vi "Set Auxiliary Amplifier Mode.vi"(8 "error in (no error)":errorcluster, 10 "Amplifier Mode (F: Off)":bool, 11 "VISA resource name":refnum<visa-resource-name>) -> (0 "error out":errorcluster, 3 "VISA resource name out":refnum<visa-resource-name>)   [LabVIEW 2013, in "Fluke 5XXX Series Multicalibrators.lvlib"]
doc: "This VI activate or deactivate an auxiliary amplifier and set the source preference to this amplifier or to the calibrator.\n\nNotes:\n\n(1) An error is reported if the auxiliary amplifier cannot be turned on or off for the present output.\n\n(2) Instrument model 5520A and 57LFC can not use auxiliary amplifier."
uses:
  Fluke 5XXX Series Multicalibrators.lvlib
panel:
  # "On"
  # "Off"
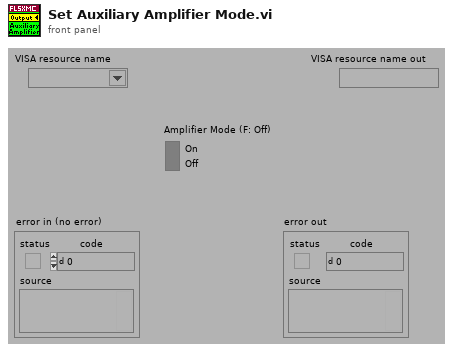
[diagram p1: front panel]
types:
  T1 = cluster{"Status":bool, "Code":i32, "Source (VI Name)":string}
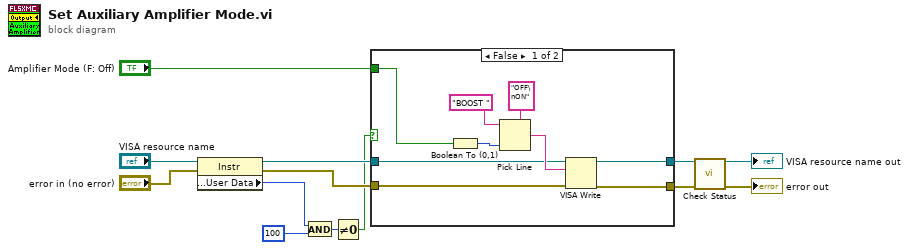
[diagram p0: block diagram]
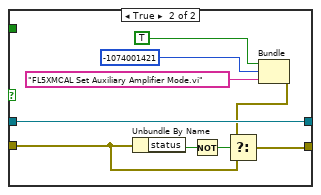
[diagram p2: hidden frame]
diagram:
  n1 = property class="Instr"(reference="VISA resource name", error in="error in (no error)") -> (reference out=w6:refnum<visa-resource-name>, error out=w5:errorcluster, "General Settings:User Data"=w4:u32)
  n2 = And(x=w4, y=u32 100 ("Numeric")) -> (x .and. y?=w2:u32)
  n3 = Not Equal To 0?(x=w2) -> (x != 0?=w1:bool)
  n4 = case shown="False" w1 {
    tunnel: "Amplifier Mode (F: Off)" -> [w19 _]
    tunnel: [w17 w28] -> w10
    tunnel: [w18 w23] -> w9
    tunnel: w6 -> [w15 w28]
    tunnel: w5 -> [w14 w25]
    frame False {
      n5 = Boolean To (0,1)(Boolean=w19) -> (0, 1=w20:i16)
      n6 = Pick Line(string ("")="BOOST " ("Reset Command"), multi-line string="OFF\nON", line index=w20) -> (output string=w16:string)
      n7 = VISA Write(VISA resource name=w15, write buffer=w16, error in (no error)=w14) -> (VISA resource name out=w17:refnum<visa-resource-name>, error out=w18:errorcluster)  [unwired: 1 out]
    }
    frame True {
      n8 = Unbundle By Name(w25) -> ("status"=w27:bool)
      n9 = Not(x=w27) -> (.not. x?=w26:bool)
      n10 = Bundle("Status"=TRUE, "Code"=-1074001421, "Source (VI Name)"="FL5XMCAL Set Auxiliary Amplifier Mode.vi") -> (w24:T1)  [unwired: 1 in]
      n11 = Select(t=w24, s=w26, f=w25) -> (s? t:f=w23:errorcluster)
    }
  }
  n12 = call "Check Status.vi"("VISA resource name"=w10, "error in (no error)"=w9) -> ("VISA resource name out"=→"VISA resource name out":refnum<visa-resource-name>, "error out"=→"error out":errorcluster)  [unwired: 12 in]
